vi "voltageToTemp.vi"(0 "waveform":waveform(dbl)) -> (1 "rawVoltage":dbl, 2 "degC":dbl)   [LabVIEW 2018]
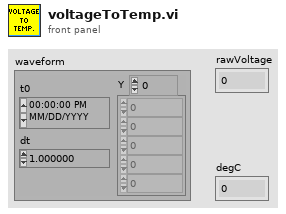
[diagram p1: front panel]
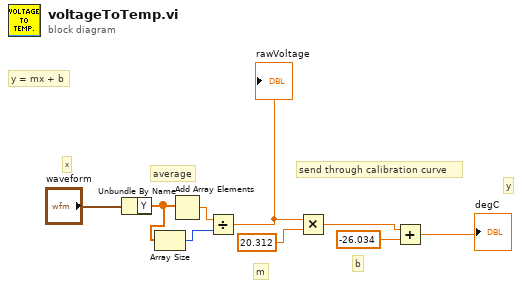
[diagram p0: block diagram]
diagram:
  # "y"
  # "x"
  # "y = mx + b"
  # "m"
  # "b"
  # "send through calibration curve"
  # "average"
  n1 = Unbundle By Name("waveform") -> ("Y"=w6:dbl[])
  n2 = Array Size(array=w6) -> (size(s)=w8:i32)
  n3 = Add Array Elements(numeric array=w6) -> (sum=w9:dbl)
  n4 = Divide(x=w9, y=w8) -> (x/y=w3:dbl)
  "rawVoltage" <- w3
  n5 = Multiply(x=w3, y=20.312) -> (x*y=w1:dbl)
  n6 = Add(x=w1, y=-26.034) -> (x+y=→"degC":dbl)
